vi "Write Default Headers.vi"(8 "error in (no error)":errorcluster, 10 "Headers":cluster{"header":string, "value":string}[](array[cluster]), 11 "REST Client in":refnum<class "REST Client.lvclass">) -> (0 "error out":errorcluster, 3 "REST Client out":refnum<class "REST Client.lvclass">)   [LabVIEW 2013, in "REST Client.lvlib" / "REST Client.lvclass"]
doc: "Write Default Headers"
uses:
  REST Client.lvclass
  REST Client.lvclass/REST Client.ctl
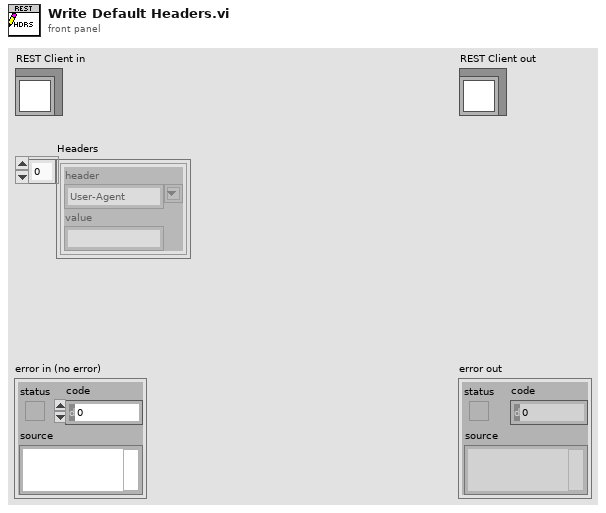
[diagram p1: front panel]
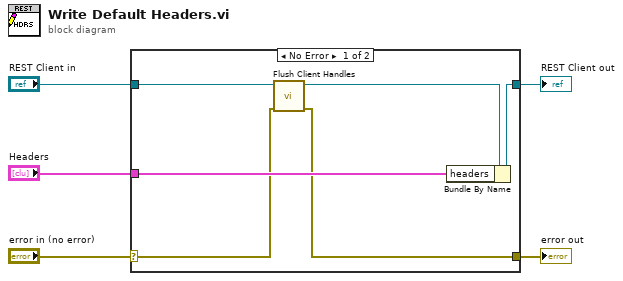
[diagram p0: block diagram]
diagram:
  n1 = case shown="No Error" "error in (no error)" {
    selector: "error in (no error)" -> [w7 w12]
    tunnel: [w6 w12] -> w4
    tunnel: [w11 w13] -> w2
    tunnel: "REST Client in" -> [w9 w13]
    tunnel: "Headers" -> [w10 _]
    frame No Error {
      n2 = call-dynamic "Flush Client Handles.vi"("error in (no error)"=w7, "REST Client in"=w9) -> ("error out"=w6:errorcluster, "REST Client out"=w8:refnum<class "REST Client.lvclass">)  [unwired: 8 in]
      n3 = Bundle By Name(cluster=w8, "headers"=w10) -> (w11:refnum<class "REST Client.lvclass">)
    }
    frame Error {
    }
  }
  "error out" <- w4
  "REST Client out" <- w2
